vi "take image.vi"(6 "Voltage":dbl, 7 "Exposure time":dbl, 8 "expose any":refnum<k21>, 9 "Busy out":refnum<k21>, 10 "Exp In":refnum<k21>, 11 "Galvo":refnum<k21>) -> ()   [LabVIEW 2021]
uses:
  <vilib>/DAQmx/write.llb/DAQmx Write (Digital Bool 1Line 1Point).vi
  <vilib>/DAQmx/read.llb/DAQmx Read (Digital Bool 1Line 1Point).vi
  <vilib>/DAQmx/write.llb/DAQmx Write (Analog DBL 1Chan 1Samp).vi
  <vilib>/DAQmx/miscellaneous.llb/DAQmx Fill In Error Info.vi
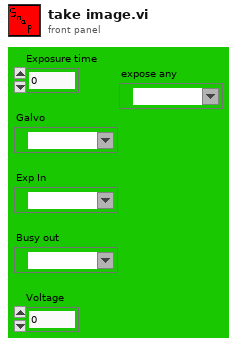
[diagram p1: front panel]
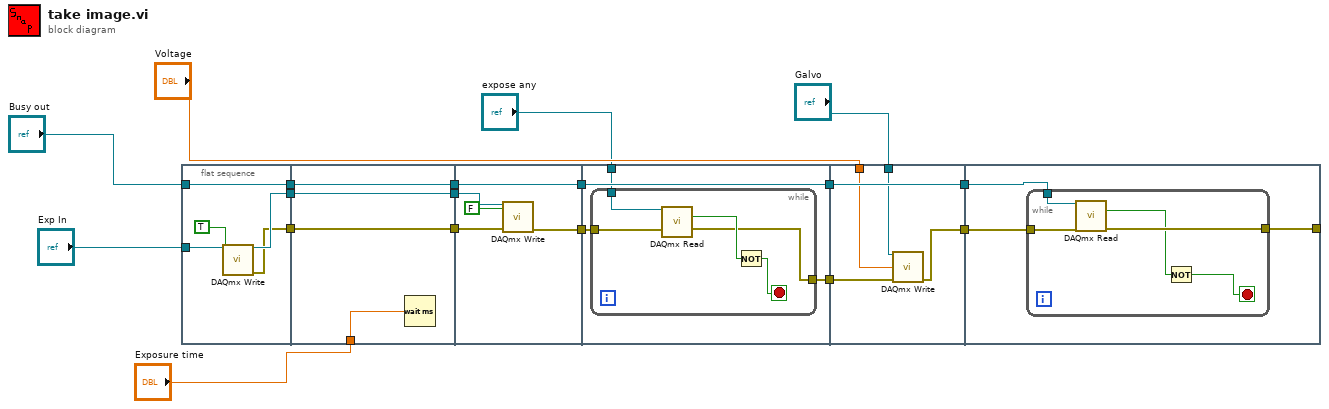
[diagram p0: block diagram]
diagram:
  n1 = flat-sequence {
    tunnel: [w22] -> w18
    tunnel: [w21] -> w17
    tunnel: "Busy out" -> [w20]
    tunnel: [w20] -> w16
    tunnel: "Exp In" -> [w19]
    tunnel: w18 -> [w27]
    tunnel: [w27] -> w15
    tunnel: w17 -> [w25]
    tunnel: [w26] -> w14
    tunnel: w16 -> [w26]
    tunnel: [w25] -> w13
    tunnel: "Exposure time" -> [w24]
    tunnel: w15 -> [w32]
    tunnel: [w30] -> w7
    tunnel: w14 -> [w30]
    tunnel: w13 -> [w29]
    tunnel: [w28] -> w6
    tunnel: w7 -> [w36]
    tunnel: [w36] -> w4
    tunnel: w6 -> [w34]
    tunnel: "expose any" -> [w35]
    tunnel: [w33] -> w3
    tunnel: w4 -> [w46]
    tunnel: [w46] -> w2
    tunnel: [w43] -> w1
    tunnel: "Voltage" -> [w45]
    tunnel: "Galvo" -> [w44]
    tunnel: w3 -> [w42]
    tunnel: w2 -> [w49]
    tunnel: w1 -> [w48]
    tunnel: [w47] -> _
    frame #0 {
      n2 = call-poly <vilib>:"DAQmx Write.vi"("task/channels in"=w19, "data"=TRUE) -> ("task out"=w22:refnum<k21>, "error out"=w21:errorcluster)  [unwired: 11 in, 1 out]
    }
    frame #1 {
      n3 = Wait (ms)(milliseconds to wait=w24) -> ()  [unwired: 1 out]
    }
    frame #2 {
      n4 = call-poly <vilib>:"DAQmx Write.vi"("task/channels in"=w32, "data"=FALSE, "error in"=w29) -> ("error out"=w28:errorcluster)  [unwired: 10 in, 2 out]
    }
    frame #3 {
      n5 = while {
        tunnel: w35 -> [w41]
        tunnel: w34 -> [w38]
        tunnel: [w37] -> w33
        stop <- w39 stop-if-true
        n6 = call-poly <vilib>:"DAQmx Read.vi"("task/channels in"=w41, "error in"=w38) -> ("data"=w40:bool, "error out"=w37:errorcluster)  [unwired: 11 in, 1 out]
        n7 = Not(x=w40) -> (.not. x?=w39:bool)
      }
    }
    frame #4 {
      n8 = call-poly <vilib>:"DAQmx Write.vi"("task/channels in"=w44, "data"=w45, "error in"=w42) -> ("error out"=w43:errorcluster)  [unwired: 10 in, 2 out]
    }
    frame #5 {
      n9 = while {
        tunnel: w49 -> [w54]
        tunnel: w48 -> [w53]
        tunnel: [w52] -> w47
        stop <- w51 stop-if-true
        n10 = call-poly <vilib>:"DAQmx Read.vi"("task/channels in"=w54, "error in"=w53) -> ("data"=w50:bool, "error out"=w52:errorcluster)  [unwired: 11 in, 1 out]
        n11 = Not(x=w50) -> (.not. x?=w51:bool)
      }
    }
  }
